vi "test Counter.vi"(8 "error in (no error)":errorcluster, 11 "TestCase in":refnum<class "Scan Engine cRIO System Tests.lvclass">) -> (0 "error out":errorcluster, 3 "TestCase out":refnum<class "Scan Engine cRIO System Tests.lvclass">)   [LabVIEW 2016, in "Scan Engine cRIO System Tests.lvclass"]
uses:
  Scan Engine cRIO System Tests.lvclass
  C:/Users/rzoeller/Documents/ni-official/niveristand-custom-device-testing-tools/VeriStandTestCase/VeriStandTestCase.lvclass
  <vilib>/NI Veristand/Execution/Workspace/NI VeriStand - Get Single Channel Value.vi
  <vilib>/addons/_JKI Toolkits/VI Tester/TestCase.llb/TestCase.lvclass
  <vilib>/NI VeriStand/Execution/Workspace/NI_VS Workspace ExecutionAPI.lvlib
  C:/Program Files (x86)/National Instruments/LabVIEW 2016/vi.lib/addons/_JKI Toolkits/VI Tester/TestCase.llb/TestCase.lvclass
panel:
  in  "Terminal Count":i32=10
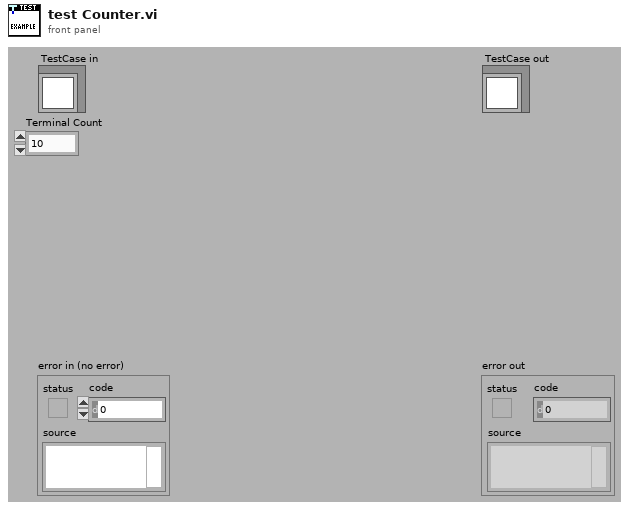
[diagram p1: front panel]
types:
  T1 = typedef "NI_VS Workspace ExecutionAPI.lvlib/WorkspaceAPI.ctl" = refnum<k24>
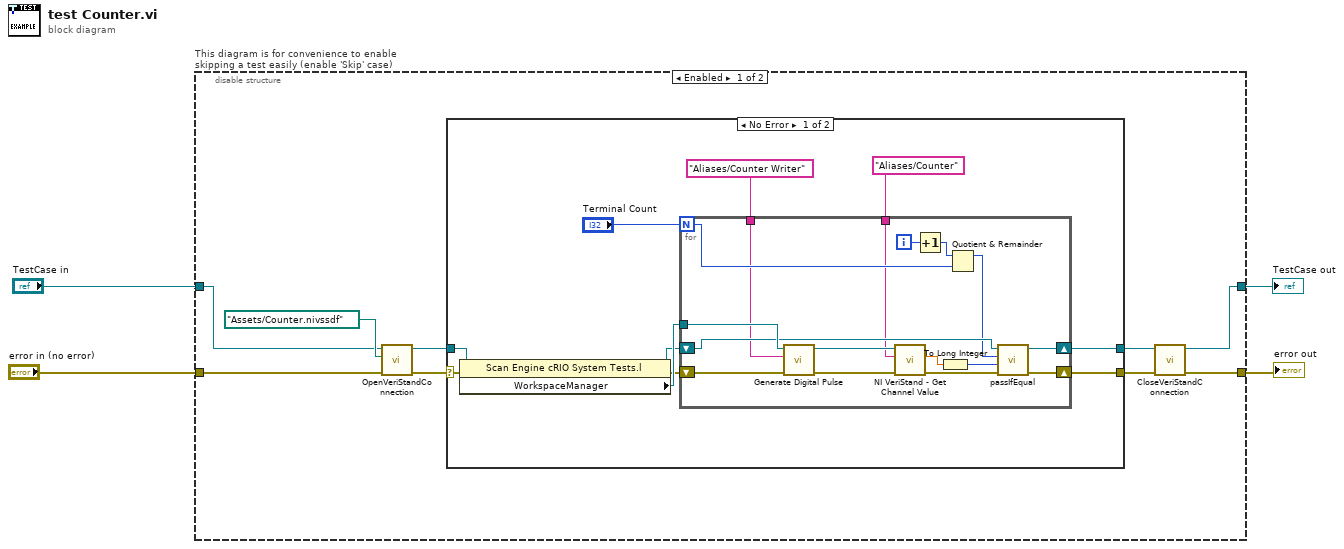
[diagram p0: block diagram]
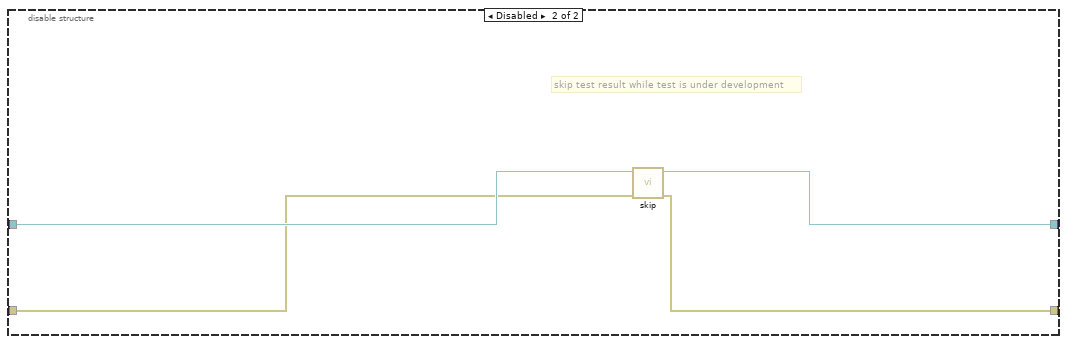
[diagram p3: hidden frame]
diagram:
  n1 = disable-structure "This diagram is for convenience to enable skipping a test easily (enable 'Skip' case)" shown="Enabled" {
    disable-tunnel: "TestCase in" -> [w9 w45]
    disable-tunnel: [w5 w43] -> w1
    disable-tunnel: [w7 w44] -> w3
    disable-tunnel: "error in (no error)" -> [w11 w42]
    frame Enabled {
      n2 = call-dynamic "OpenVeriStandConnection.vi"("error in (no error)"=w11, "System Definition File"=path "Assets/Counter.nivssdf", "VeriStand Test Case in"=w9) -> ("error out"=w12:errorcluster, "VeriStand Test Case out"=w10:refnum<class "Scan Engine cRIO System Tests.lvclass">)  [unwired: 7 in]
      n3 = case shown="No Error" w12 {
        selector: w12 -> [w16 w41]
        tunnel: [w20 w41] -> w8
        tunnel: [w14 w40] -> w6
        tunnel: w10 -> [w15 w40]
        frame No Error {
          n4 = property class="Scan Engine cRIO System Tests.l"(reference=w15, error in=w16) -> (reference out=w19:refnum<class "Scan Engine cRIO System Tests.lvclass">, error out=w22:errorcluster, "WorkspaceManager"=w23:T1)
          n5 = for {
            N: "Terminal Count" -> [w27]
            tunnel: w23 -> [w39]
            shift-right: [w34] -> w20
            shift-left: w22 -> [w38]
            shift-right: [w31] -> w14
            shift-left: w19 -> [w32]
            tunnel: "Aliases/Counter" ("Channel") -> [w25]
            tunnel: "Aliases/Counter Writer" ("Channel") -> [w24]
            i -> [w33]
            n6 = call "Generate Digital Pulse.vi"("error in (no error)"=w38, "Channel"=w24, "WorkspaceManager"=w39) -> ("error out"=w37:errorcluster, "Workspace Manager out"=w36:T1)  [unwired: 7 in]
            n7 = call-poly <vilib>:"NI VeriStand - Get Channel Value.vi"("error in (no error)"=w37, "Channel"=w25, "WorkspaceManager in"=w36) -> ("error out"=w35:errorcluster, "Value"=w29:dbl)  [unwired: 6 in, 1 out]
            n8 = Increment(x=w33) -> (x+1=w28:i32)
            n9 = To Long Integer(number=w29) -> (32bit integer=w30:i32)
            n10 = Quotient & Remainder(x=w28, y=w27) -> (x-y*floor(x/y)=w26:i32)  [unwired: 1 out]
            n11 = call-dynamic "passIfEqual.vi"("error in (no error)"=w35, "y"=w30, "x"=w26, "TestCase in"=w32) -> ("error out"=w34:errorcluster, "TestCase out"=w31:refnum<class "Scan Engine cRIO System Tests.lvclass">)  [unwired: 6 in]
          }
        }
        frame Error {
        }
      }
      n12 = call-dynamic "CloseVeriStandConnection.vi"("error in (no error)"=w8, "VeriStand Test Case in"=w6) -> ("error out"=w7:errorcluster, "VeriStand Test Case out"=w5:refnum<class "Scan Engine cRIO System Tests.lvclass">)  [unwired: 8 in]
    }
    frame Disabled {
      # "skip test result while test is under development"
      n13 = call <vilib>:"skip.vi"("error in (no error)"=w42, "TestCase in"=w45) -> ("error out"=w44:errorcluster, "TestCase out"=w43:refnum<class "Scan Engine cRIO System Tests.lvclass">)  [unwired: 8 in]
    }
  }
  "error out" <- w3
  "TestCase out" <- w1
